vi "sedSpectrometer_getEvent_MeasuredSpectrum.vi"(8 "error in (no error)":errorcluster, 11 "logevent_MeasuredSpectrum_Ctl":T1={"spectId"=0, "wavelength[2048]"=array[2048 elements], "intensity[2048]"=array[2048 elements], "imageName"="", "frameNumber"=0, "pixelNumber"=0, "exposureStartTime"=0.0, "exposureLength"=0, "SpectSNo"="", "SpectTemp"=0, "CommandedTemp"=0, "priority"=0}) -> (0 "error out":errorcluster, 2 "function return":i32, 3 "logevent_MeasuredSpectrum_Ctl out":T1)   [LabVIEW 2016, in "SALLV_sedSpectrometer.lvlib"]
doc: "int sedSpectrometer_shm_getEvent_MeasuredSpectrumLV(sedSpectrometer_logevent_MeasuredSpectrumLV *logevent_MeasuredSpectrum_Ctl );"
uses:
  SALLV_sedSpectrometer.lvlib
  DataTypes/logevent_MeasuredSpectrum.ctl
  SALLV_sedSpectrometer.so
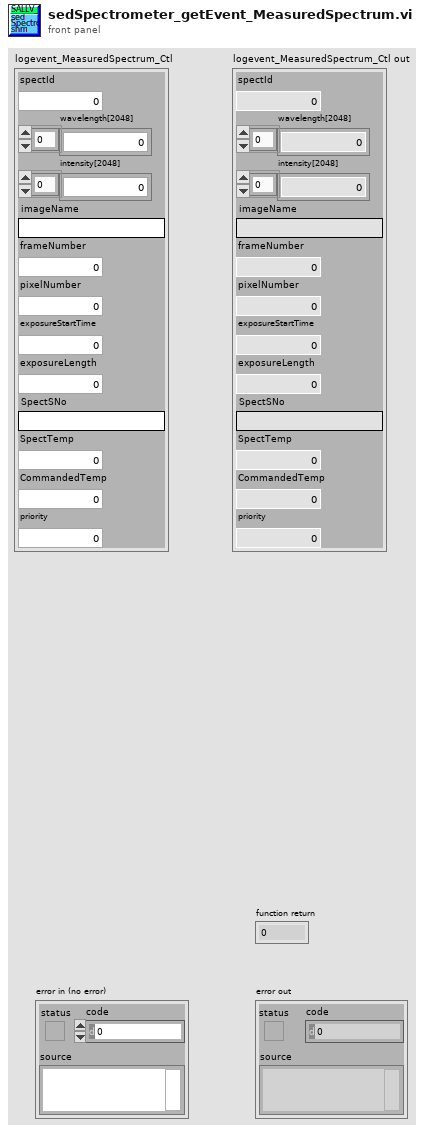
[diagram p1: front panel]
types:
  T1 = typedef "SALLV_sedSpectrometer.lvlib/logevent_MeasuredSpectrum.ctl" = cluster{"spectId":u16, "wavelength[2048]":dbl[], "intensity[2048]":dbl[], "imageName":string, "frameNumber":i32, "pixelNumber":u32, "exposureStartTime":dbl, "exposureLength":i32, "SpectSNo":string, "SpectTemp":i32, "CommandedTemp":i32, "priority":i32}
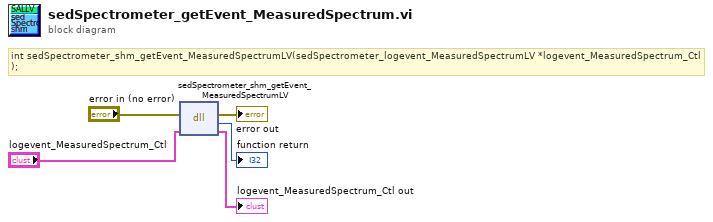
[diagram p0: block diagram]
diagram:
  # "int sedSpectrometer_shm_getEvent_MeasuredSpectrumLV(sedSpectrometer_logevent_MeasuredSpectrumLV *logevent_MeasuredSpectrum_Ctl );"
  n1 = dll-call lib="home/harini/TCS/SALLV_sedSpectrometer/SALLV_sedSpectrometer.*" fn="sedSpectrometer_shm_getEvent_MeasuredSpectrumLV"(error in="error in (no error)", "logevent_MeasuredSpectrum_Ctl"="logevent_MeasuredSpectrum_Ctl") -> (error out=→"error out":errorcluster, →"function return":i32, "logevent_MeasuredSpectrum_Ctl"=→"logevent_MeasuredSpectrum_Ctl out":T1)  [unwired: 2 in, 1 out]
